vi "DTFT (SubVI).vi"(11 "ip array":dbl[](array[numeric])) -> (2 "Magnitude op":dbl[](array[numeric]), 3 "DTFT op":cdb[](array[numeric]))   [LabVIEW 2014]
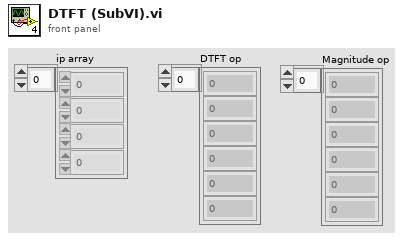
[diagram p1: front panel]
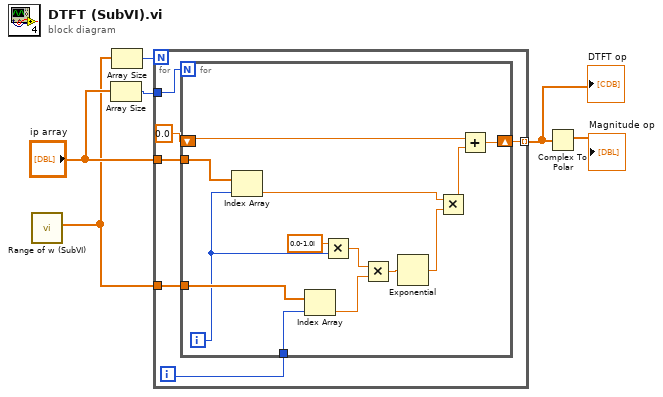
[diagram p0: block diagram]
diagram:
  n1 = call "Range of w (SubVI).vi"() -> ("-pi to pi"=w2:dbl[])  [unwired: 11 in]
  n2 = Array Size(array="ip array") -> (size(s)=w3:i32)
  n3 = Array Size(array=w2) -> (size(s)=w1:i32)
  n4 = for {
    N: w1 -> [_]
    tunnel: w2 -> [w11]
    tunnel: w3 -> [w10]
    tunnel: "ip array" -> [w8]
    tunnel: [w7] -> w4 mode=indexing
    i -> [w12]
    n5 = for {
      N: w10 -> [_]
      tunnel: w12 -> [w24]
      tunnel: w11 -> [w23]
      shift-right: [w17] -> w7
      shift-left: 0.0 -> [w16]
      tunnel: w8 -> [w13]
      i -> [w14]
      n6 = Index Array(array=w13, index=w14) -> (element=w15:dbl)
      n7 = Index Array(array=w23, index=w24) -> (element=w21:dbl)
      n8 = Multiply(x=cdb 0.0-1.0i, y=w14) -> (x*y=w22:cdb)
      n9 = Multiply(x=w22, y=w21) -> (x*y=w20:cdb)
      n10 = Exponential(1:w20) -> (0:w19:cdb)
      n11 = Multiply(x=w15, y=w19) -> (x*y=w18:cdb)
      n12 = Add(x=w16, y=w18) -> (x+y=w17:cdb)
    }
  }
  "DTFT op" <- w4
  n13 = Complex To Polar(r * e^(i*theta)=w4) -> (r=→"Magnitude op":dbl[])  [unwired: 1 out]
